vi "Prime BSI Camera Messenger.vi"(0 "Notifier Name":string, 2 "Prime Actions":T5, 5 "Prime Parameter":T2, 7 "ROI Setup":T1, 9 "# of Frames":u32, 11 "Error In":errorcluster, 12 "File Save Path":path) -> (4 "Notifier Name (Dup)":string, 6 "Prime Parameter":T2, 8 "Prime ROI":T1, 10 "Running?":bool, 13 "Image Ref":T4, 15 "Error Out":errorcluster)   [LabVIEW 2025]
uses:
  Prime BSI Type Defs/Prime BSI Actions.ctl
  Prime BSI Type Defs/Prime BSI Parameters.ctl
  Prime BSI Type Defs/Prime BSI Parameter List.ctl
  Prime BSI Type Defs/Prime BSI ROI.ctl
  <vilib>/vision/Image Controls.llb/IMAQ Image.ctl
  Prime BSI Type Defs/Prime BSI Notifier Element.ctl
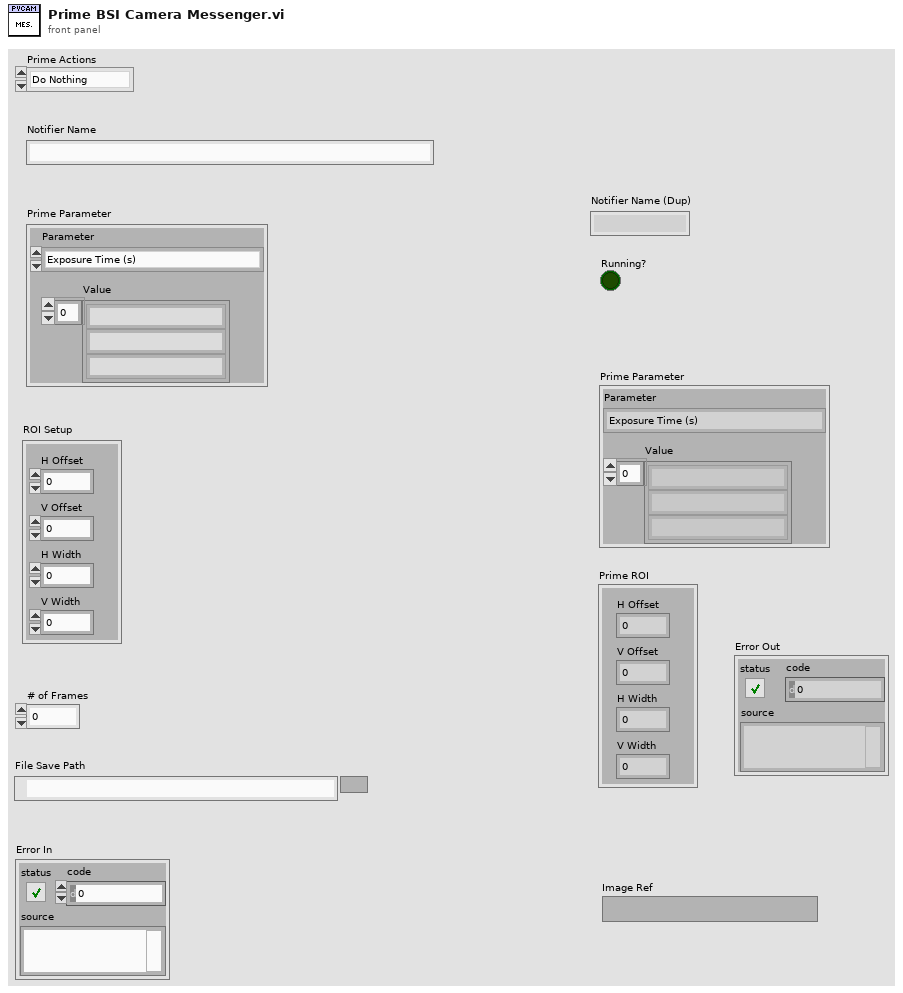
[diagram p1: front panel]
types:
  T1 = typedef "Prime BSI ROI.ctl" = cluster{"H Offset":i32, "V Offset":i32, "H Width":i32, "V Width":i32}
  T2 = typedef "Prime BSI Parameters.ctl" = cluster{"Parameter":T3, "Value":string[]}
  T3 = typedef "Prime BSI Parameter List.ctl" = enum16{"Exposure Time (s)", "Binning", "Readout Port List", "Available Gain List"}
  T4 = typedef "IMAQ Image.ctl" = refnum<image>
  T5 = typedef "Prime BSI Actions.ctl" = enum16{"Do Nothing", "Preview", "Record", "Abort", "Record Settings", "Set Parameter", "Get Parameter", "Set ROI", "Get ROI", "Status", "Quit"}
  T6 = typedef "Prime BSI Notifier Element.ctl" = cluster{"PVCam Actions":T5, "Received?":bool, "PVCam Parameter":T2, "PVCam ROI":T1, "Running?":bool, "File Path":path, "# of frames":u32, "Image Ref":T4, "Binning":i32}
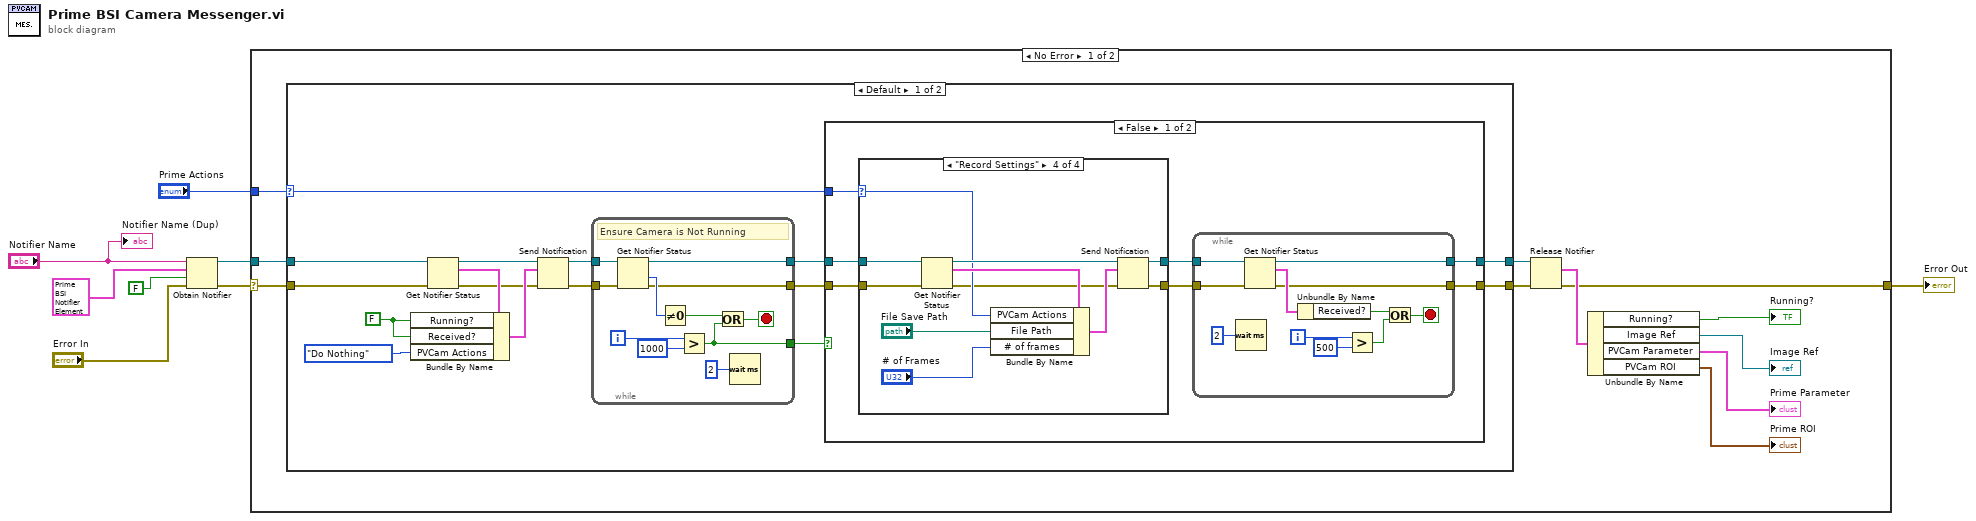
[diagram p0: block diagram]
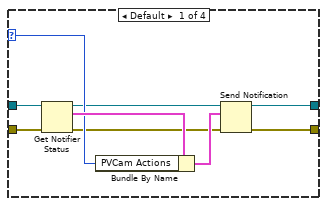
[diagram p2: hidden frame]
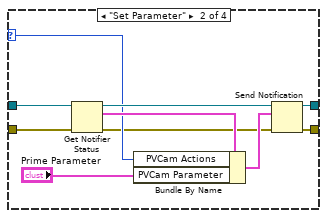
[diagram p3: hidden frame]
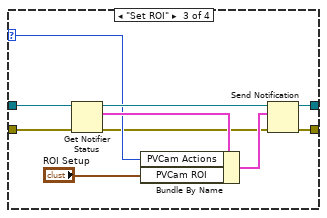
[diagram p4: hidden frame]
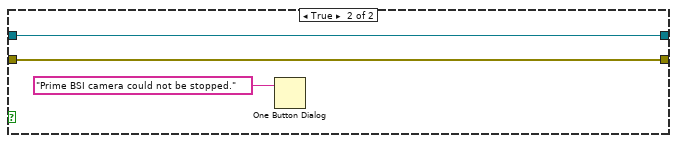
[diagram p5: hidden frame]
diagram:
  n1 = Obtain Notifier(name (unnamed)="Notifier Name", notification data type=T6 {"PVCam Actions"=enum."Do Nothing", "Received?"=FALSE, "PVCam Parameter"={"Parameter"=enum."Exposure Time (s)", "Value"=[]}, "PVCam ROI"={"H Offset"=0, "V Offset"=0, "H Width"=0, "V Width"=0}, "Running?"=FALSE, "File Path"=path "", "# of frames"=0, "Image Ref"=refnum, "Binning"=0} ("Prime Camera Cluster"), create if not found? (T)=FALSE, error in (no error)="Error In") -> (notifier out=w6:refnum<notifier>, error out=w7:errorcluster)  [unwired: 1 out]
  n2 = case shown="No Error" w7 {
    selector: w7 -> [w11 w110]
    tunnel: w6 -> [w19 _]
    tunnel: "Prime Actions" -> [w18 _]
    tunnel: [w9 w110] -> w1
    frame No Error {
      n3 = case shown="Default" w18 {
        selector: w18 -> [w31 _]
        tunnel: w19 -> [w35 w109]
        tunnel: [w30 w109] -> w13
        tunnel: w11 -> [w25 w108]
        tunnel: [w21 w108] -> w10
        frame Default {
          w26 = FALSE ("Running?")
          n4 = Get Notifier Status(notifier=w35, error in (no error)=w25) -> (notifier out=w29:refnum<notifier>, current notification=w28:T6, error out=w24:errorcluster)  [unwired: 2 out]
          n5 = Bundle By Name(cluster=w28, "Running?"=w26, "Received?"=w26, "PVCam Actions"=Prime_BSI_Actions."Do Nothing") -> (w27:T6)
          n6 = Send Notification(notification=w27, notifier=w29, error in (no error)=w24) -> (notifier out=w34:refnum<notifier>, error out=w23:errorcluster)
          n7 = while {
            tunnel: w34 -> [w107]
            tunnel: [w106] -> w32
            tunnel: [w101] -> w33
            tunnel: w23 -> [w99]
            tunnel: [w97] -> w22
            i -> [w103]
            stop <- w105 stop-if-true
            # "Ensure Camera is Not Running"
            n8 = Get Notifier Status(notifier=w107, error in (no error)=w99) -> (notifier out=w106:refnum<notifier>, # waiting=w98:i32, error out=w97:errorcluster)  [unwired: 2 out]
            n9 = Not Equal To 0?(x=w98) -> (x != 0?=w100:bool)
            n10 = Greater?(x=w103, y=1000) -> (0:w101:bool)
            n11 = Or(x=w100, y=w101) -> (x .or. y?=w105:bool)
            n12 = Wait (ms)(milliseconds to wait=u32 2) -> ()  [unwired: 1 out]
          }
          n13 = case shown="False" w33 {
            tunnel: w32 -> [w40 w95]
            tunnel: w31 -> [w42 _]
            tunnel: [w39 w95] -> w30
            tunnel: w22 -> [w38 w94]
            tunnel: [w36 w94] -> w21
            frame False {
              n14 = case shown="\"Record Settings\"" w42 {
                selector: w42 -> [w60 w67 w77 w88]
                tunnel: w40 -> [w62 w72 w82 w93]
                tunnel: [w58 w70 w80 w91] -> w41
                tunnel: w38 -> [w56 w65 w75 w85]
                tunnel: [w54 w63 w73 w83] -> w37
                frame Default {
                  n15 = Get Notifier Status(notifier=w62, error in (no error)=w56) -> (notifier out=w59:refnum<notifier>, current notification=w61:T6, error out=w55:errorcluster)  [unwired: 2 out]
                  n16 = Bundle By Name(cluster=w61, "PVCam Actions"=w60) -> (w57:T6)
                  n17 = Send Notification(notification=w57, notifier=w59, error in (no error)=w55) -> (notifier out=w58:refnum<notifier>, error out=w54:errorcluster)
                }
                frame "Set Parameter" {
                  n18 = Get Notifier Status(notifier=w72, error in (no error)=w65) -> (notifier out=w71:refnum<notifier>, current notification=w69:T6, error out=w64:errorcluster)  [unwired: 2 out]
                  n19 = Bundle By Name(cluster=w69, "PVCam Actions"=w67, "PVCam Parameter"="Prime Parameter") -> (w68:T6)
                  n20 = Send Notification(notification=w68, notifier=w71, error in (no error)=w64) -> (notifier out=w70:refnum<notifier>, error out=w63:errorcluster)
                }
                frame "Set ROI" {
                  n21 = Get Notifier Status(notifier=w82, error in (no error)=w75) -> (notifier out=w81:refnum<notifier>, current notification=w79:T6, error out=w74:errorcluster)  [unwired: 2 out]
                  n22 = Bundle By Name(cluster=w79, "PVCam Actions"=w77, "PVCam ROI"="ROI Setup") -> (w78:T6)
                  n23 = Send Notification(notification=w78, notifier=w81, error in (no error)=w74) -> (notifier out=w80:refnum<notifier>, error out=w73:errorcluster)
                }
                frame "Record Settings" {
                  n24 = Get Notifier Status(notifier=w93, error in (no error)=w85) -> (notifier out=w92:refnum<notifier>, current notification=w90:T6, error out=w84:errorcluster)  [unwired: 2 out]
                  n25 = Bundle By Name(cluster=w90, "PVCam Actions"=w88, "File Path"="File Save Path", "# of frames"="# of Frames") -> (w89:T6)
                  n26 = Send Notification(notification=w89, notifier=w92, error in (no error)=w84) -> (notifier out=w91:refnum<notifier>, error out=w83:errorcluster)
                }
              }
              n27 = while {
                tunnel: w41 -> [w53]
                tunnel: [w45] -> w39
                tunnel: w37 -> [w44]
                tunnel: [w43] -> w36
                i -> [w50]
                stop <- w46 stop-if-true
                n28 = Wait (ms)(milliseconds to wait=u32 2) -> ()  [unwired: 1 out]
                n29 = Get Notifier Status(notifier=w53, error in (no error)=w44) -> (notifier out=w45:refnum<notifier>, current notification=w52:T6, error out=w43:errorcluster)  [unwired: 2 out]
                n30 = Unbundle By Name(w52) -> ("Received?"=w51:bool)
                n31 = Greater?(x=w50, y=500) -> (0:w48:bool)
                n32 = Or(x=w51, y=w48) -> (x .or. y?=w46:bool)
              }
            }
            frame True {
              n33 = One Button Dialog(message="Prime BSI camera could not be stopped.") -> ()  [unwired: 1 in, 1 out]
            }
          }
        }
        frame "Status" {
        }
      }
      n34 = Release Notifier(notifier=w13, error in (no error)=w10) -> (last notification=w12:T6, error out=w9:errorcluster)  [unwired: 1 in, 1 out]
      n35 = Unbundle By Name(w12) -> ("Running?"=→"Running?":bool, "Image Ref"=→"Image Ref":T4, "PVCam Parameter"=→"Prime Parameter":T2, "PVCam ROI"=→"Prime ROI":T1)
    }
    frame Error {
    }
  }
  "Error Out" <- w1
  "Notifier Name (Dup)" <- "Notifier Name"
